vi "Traverse-Main.vi"() -> ()   [LabVIEW 2017]
uses:
  Settings/Settings-Control.ctl
  TypeDefs/Trav-Command-TD.ctl
  Globals/Trav-Positon-Info.vi
panel:
  in  "Z 4":dbl
  in  "Y 4":dbl
  in  "X 4":dbl
  in  "Trav Command":T1 items=["Set Reference", "Read Position", "Move"]
  in  "Settings":T2
  out "Z 2":dbl
  out "Y 2":dbl
  out "X 2":dbl
  out "Z":dbl
  out "Y":dbl
  out "X":dbl
  in  "OK Button":bool
  # "relative"
  # "absolute"
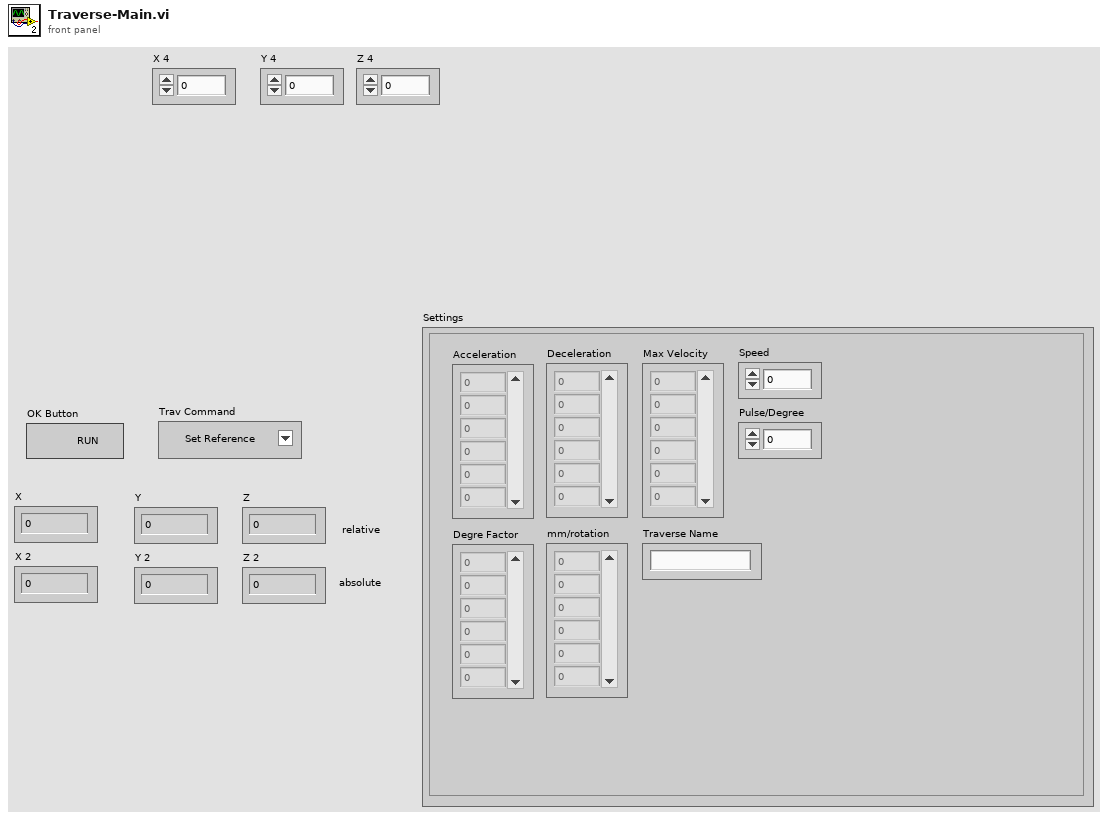
[diagram p1: front panel]
types:
  T1 = typedef "Trav-Command-TD.ctl" = u16
  T2 = typedef "Settings-Control.ctl" = cluster{"Acceleration":dbl[], "Deceleration":dbl[], "Max Velocity":dbl[], "Speed":dbl, "Pulse/Degree":dbl, "Degre Factor":dbl[], "mm/rotation":dbl[], "Traverse Name":string}
  T3 = typedef "Position-Info-TD.ctl" = cluster{"Current Position ABS":dbl[], "Current Position":dbl[], "Reference Position":dbl[], "Axis Names":string[]}
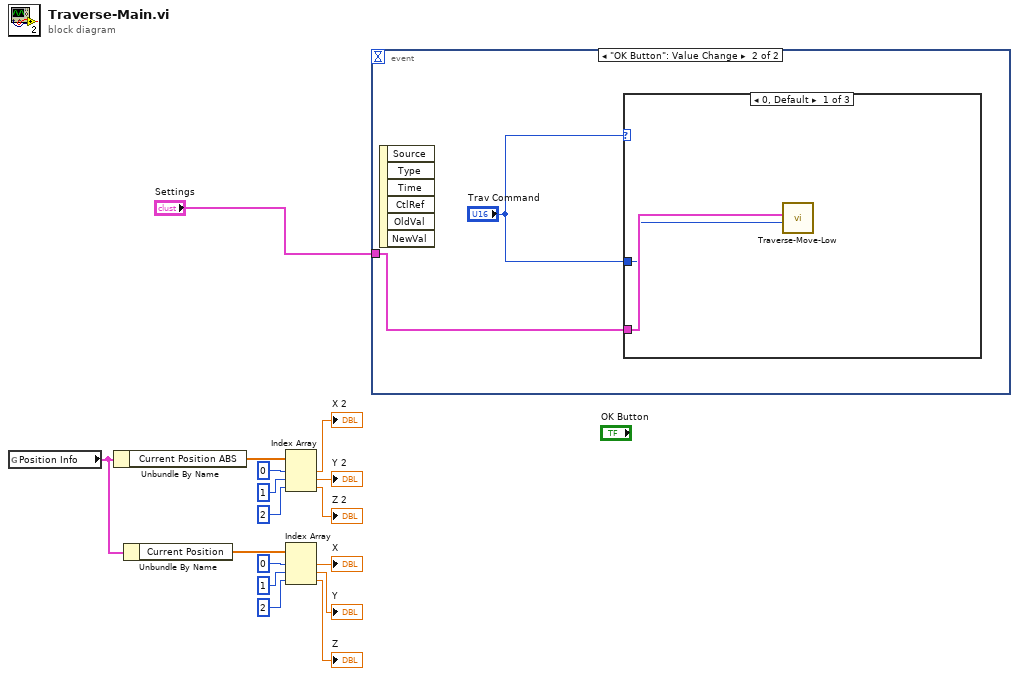
[diagram p0: block diagram]
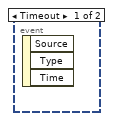
[diagram p2: hidden frame]
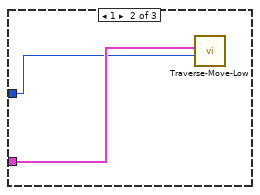
[diagram p3: hidden frame]
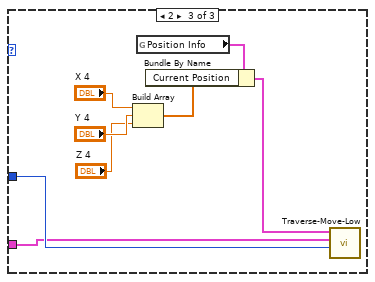
[diagram p4: hidden frame]
diagram:
  n1 = global read "Trav-Positon-Info.vi" "Position Info"() -> (w4:T3)
  n2 = Unbundle By Name(w4) -> ("Current Position ABS"=w15:dbl[])
  n3 = Unbundle By Name(w4) -> ("Current Position"=w8:dbl[])
  n4 = Index Array(array=w15, index #1=0 ("index"), index #2=1 ("index"), index #3=2 ("index")) -> (element #1=→"X 2":dbl, element #2=→"Y 2":dbl, element #3=→"Z 2":dbl)
  n5 = Index Array(array=w8, index #1=0 ("index"), index #2=1 ("index"), index #3=2 ("index")) -> (element #1=→"X":dbl, element #2=→"Y":dbl, element #3=→"Z":dbl)
  n6 = event shown="[1] \"OK Button\": Value Change" {
    selector: _ -> [_ _]
    dyn-events: _ -> [_ _]
    timeout: _ -> [_ _]
    tunnel: "Settings" -> [_ w18]
    event Timeout {
      n7 = event-data() -> ()  [unwired: 1 in, 3 out]
    }
    event "OK Button": Value Change {
      n8 = event-data() -> ()  [unwired: 1 in, 6 out]
      n9 = case shown="0, Default" "Trav Command" {
        tunnel: w18 -> [w20 w22 w23]
        tunnel: "Trav Command" -> [w19 w21 w24]
        frame 0, Default {
          n10 = call "Traverse-Move-Low.vi"("Trav Command"=w19, "Settings"=w20) -> ()  [unwired: 8 in, 2 out]
        }
        frame 1 {
          n11 = call "Traverse-Move-Low.vi"("Trav Command"=w21, "Settings"=w22) -> ()  [unwired: 8 in, 2 out]
        }
        frame 2 {
          n12 = Build Array("X 4", "Y 4", "Z 4") -> (w26:dbl[])
          n13 = global read "Trav-Positon-Info.vi" "Position Info"() -> (w25:T3)
          n14 = Bundle By Name(cluster=w25, "Current Position"=w26) -> (w27:T3)
          n15 = call "Traverse-Move-Low.vi"("Trav Command"=w24, "Settings"=w23, "Position Info IN"=w27) -> ()  [unwired: 7 in, 2 out]
        }
      }
    }
  }
